vi "DataStream_RT_Get Status.vi"(8 "Error":errorcluster, 11 "Stream Writer Ref":T1) -> (0 "Error Out":errorcluster, 1 "Writable Out":bool, 2 "Connected Out":bool, 3 "Stream Writer Ref Out":T1, 4 "RemoteEndptDestroyed Out":bool)   [LabVIEW 2023]
uses:
  TypeDefs/Cluster_DataStream_RT Writer Refs.ctl
  <resource>/objmgr/ni.dex.rc
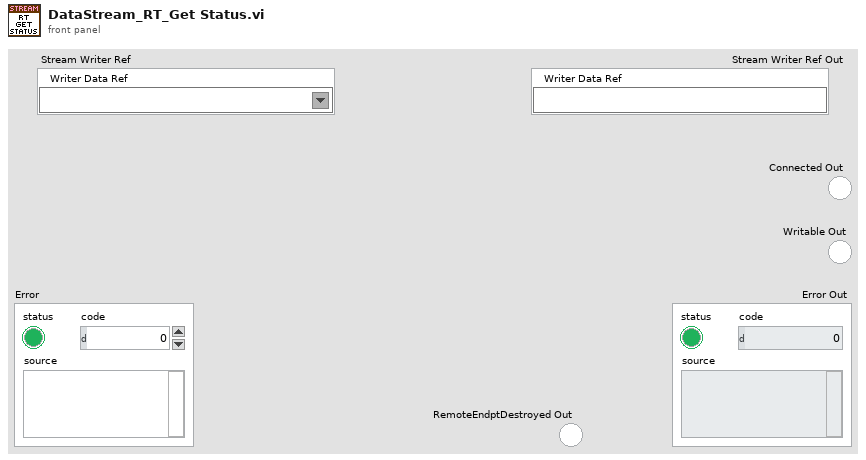
[diagram p1: front panel]
types:
  T1 = typedef "Cluster_DataStream_RT Writer Refs.ctl" = cluster{"Writer Data Ref":refnum<k21>}
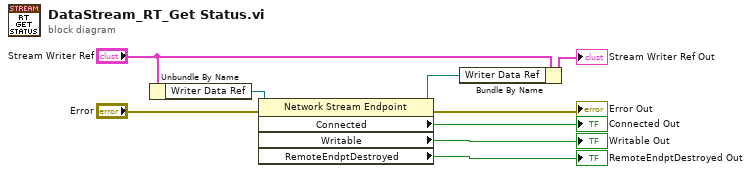
[diagram p0: block diagram]
diagram:
  n1 = Unbundle By Name("Stream Writer Ref") -> ("Writer Data Ref"=w5:refnum<k21>)
  n2 = property class="Network Stream Endpoint"(reference=w5, error in="Error") -> (reference out=w9:refnum<k21>, error out=→"Error Out":errorcluster, "Connected"=→"Connected Out":bool, "Writable"=→"Writable Out":bool, "RemoteEndptDestroyed"=→"RemoteEndptDestroyed Out":bool)
  n3 = Bundle By Name(cluster="Stream Writer Ref", "Writer Data Ref"=w9) -> (→"Stream Writer Ref Out":T1)
